vi "parameterized_SomeSessionsRegistered_InitializeSessions_InitializeCalled.vi"(8 "error in":errorcluster, 9 "expected initialize-attach calls":u32, 10 "expected initialize-initialize calls":u32, 11 "initialize and close session behavior":T1) -> (0 "error out":errorcluster, 2 "result":string, 3 "pass":bool)   [LabVIEW 2020, in "MeasurementServerTests.lvlib"]
uses:
  MeasurementServerTests.lvlib
  Helpers/Fake Session Factory/Fake Session Factory.lvclass
  da6ffb6f-c1c9-4957-84dd-e9228483c454.vi
  ffc64c76-1568-41a3-8328-b9126ac9a28d.vi
  Runtime/APIs/Session Management V1/Session Reservation/Initialize and Close Session Behavior.ctl
  Runtime/APIs/Session Management V1/Session Reservation/Session Reservation.lvclass
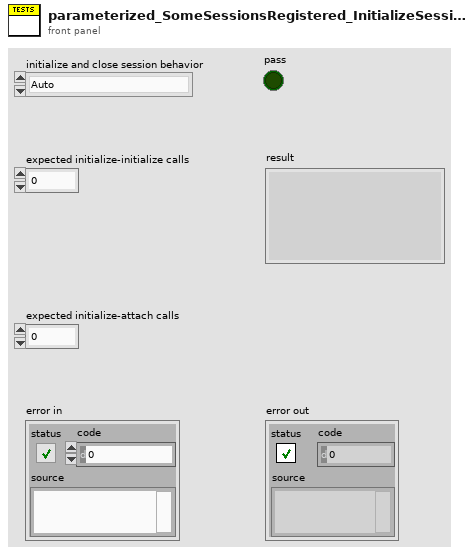
[diagram p1: front panel]
types:
  T1 = typedef "Plug-In SDK Session Management V1 API.lvlib/Session Reservation.lvclass/Initialize and Close Session Behavior.ctl" = enum16{"Auto", "Initialize and Close", "Attach and Detach", "Initialize and Detach", "Attach and Close"}
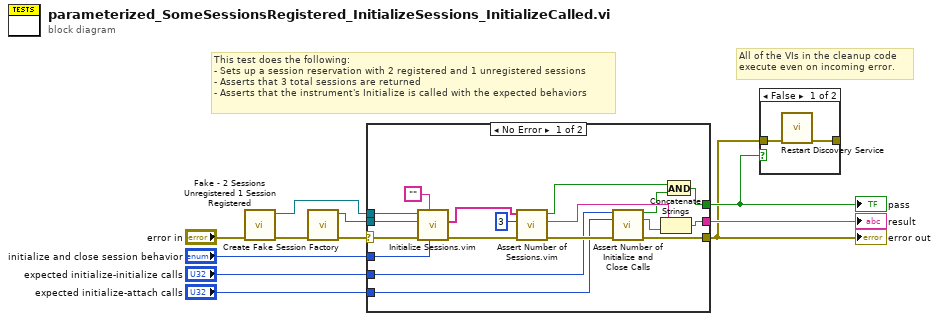
[diagram p0: block diagram]
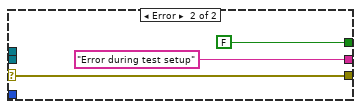
[diagram p2: hidden frame]
diagram:
  # "All of the VIs in the cleanup code\nexecute even on incoming error."
  # "This test does the following:\n- Sets up a session reservation with 2 registered and 1 unregistered sessions\n- Asserts that 3 total sessions are returned\n- Asserts that the instrument's Initialize is called with the expected behaviors"
  n1 = call "Fake - 2 Sessions Unregistered 1 Session Registered.vi"("error in"="error in") -> ("error out"=w5:errorcluster, "session reservation out"=w4:refnum<class "Session Reservation.lvclass">)  [unwired: 9 in]
  n2 = call "Create Fake Session Factory.vi"("error in"=w5) -> ("error out"=w8:errorcluster, "fake session factory out"=w7:refnum<class "Fake Session Factory.lvclass">)  [unwired: 9 in]
  n3 = case shown="No Error" w8 {
    selector: w8 -> [w27 w30]
    tunnel: [w19 w30] -> w9
    tunnel: [w18 FALSE] -> w10
    tunnel: [w16 "Error during test setup" ("f")] -> w11
    tunnel: w7 -> [w29 _]
    tunnel: w4 -> [w28 _]
    tunnel: "initialize and close session behavior" -> [w14 _]
    tunnel: "expected initialize-initialize calls" -> [w13 _]
    tunnel: "expected initialize-attach calls" -> [w12 _]
    frame No Error {
      n4 = call "Initialize Sessions.vim"("initialize and close session behavior"=w14, "session type"="", "error in"=w27, "session factory"=w29, "session reservation in"=w28) -> ("error out"=w26:errorcluster, "sessions"=w24:string[])  [unwired: 3 in, 2 out]
      n5 = call "Assert Number of Sessions.vim"("error in"=w26, "expected number of sessions"=3, "sessions"=w24) -> ("error out"=w20:errorcluster, "result"=w23:string, "pass"=w22:bool)  [unwired: 6 in]
      n6 = call "Assert Number of Initialize and Close Calls.vi"("expected initialize-initialize calls"=w13, "expected initialize-attach calls"=w12, "error in"=w20) -> ("pass"=w17:bool, "result"=w15:string, "error out"=w19:errorcluster)  [unwired: 10 in]
      n7 = Concatenate Strings(w23, w15) -> (w16:string)
      n8 = And(x=w22, y=w17) -> (x .and. y?=w18:bool)
    }
    frame Error {
    }
  }
  "error out" <- w9
  "pass" <- w10
  "result" <- w11
  n9 = case shown="False" w10 {
    tunnel: w9 -> [w34 _]
    tunnel: [w33 _] -> _
    frame False {
      n10 = call "Restart Discovery Service.vi"("error in"=w34) -> ("error out"=w33:errorcluster)  [unwired: 10 in]
    }
    frame True {
    }
  }
